vi "RS 485 COM In.vi"(8 "error in":errorcluster, 11 "9871 COM In":T1={"Data"=[0, 0, 0, 0, 0, 0, 0, 0, 0, 0, 0, 0, 0, 0, 0, 0, 0, 0, 0, 0, 0, 0, 0, 0, 0, 0, 0, 0, 0, 0], "NumBytes"=0, "Port"=enum."Port 1", "Wait for Reply"=FALSE}) -> (0 "error IO":errorcluster, 3 "9871 COM Out":T1={"Data"=[0, 0, 0, 0, 0, 0, 0, 0, 0, 0, 0, 0, 0, 0, 0, 0, 0, 0, 0, 0, 0, 0, 0, 0, 0, 0, 0, 0, 0, 0], "NumBytes"=0, "Port"=enum."Port 1", "Wait for Reply"=FALSE})   [LabVIEW 2015]
uses:
  <vilib>/eio/EIOMethodNode/EIOMethodNode.xnode
  <vilib>/rvi/eio/common/nirviEmuTemplateMethod_errors.vi
  Port Selector.ctl
  9871 COM In.ctl
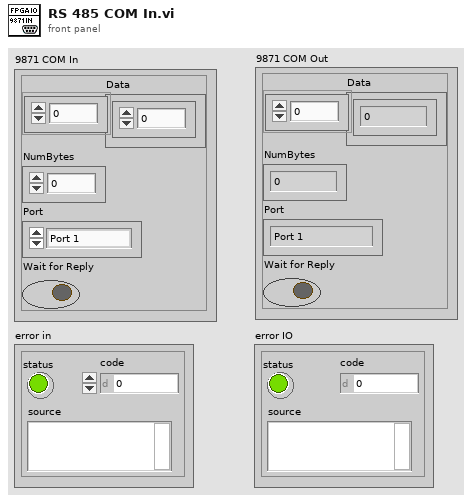
[diagram p1: front panel]
types:
  T1 = typedef "9871 COM In.ctl" = cluster{"Data":u8[], "NumBytes":i32, "Port":T2, "Wait for Reply":bool}
  T2 = typedef "Port Selector.ctl" = enum16{"Port 1", "Port 2", "Port 3", "Port 4", "None"}
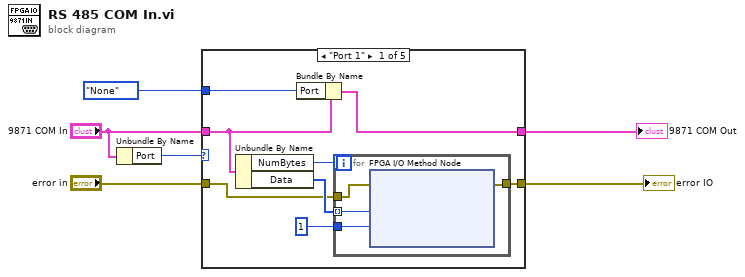
[diagram p0: block diagram]
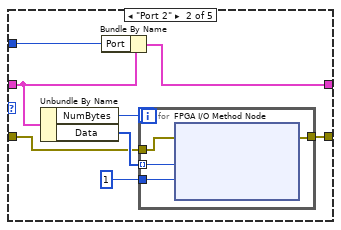
[diagram p2: hidden frame]
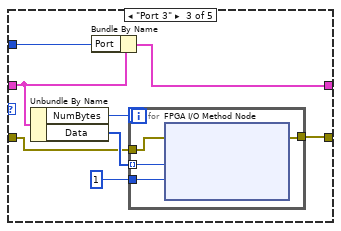
[diagram p3: hidden frame]
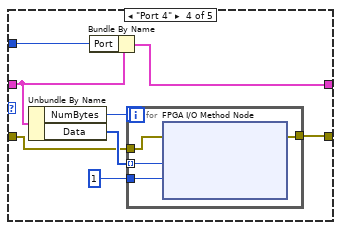
[diagram p4: hidden frame]
diagram:
  n1 = Unbundle By Name("9871 COM In") -> ("Port"=w2:T2)
  n2 = case shown="\"Port 1\"" w2 {
    tunnel: "9871 COM In" -> [w10 w26 w33 w46 w56]
    tunnel: [w11 w23 w35 w47 w56] -> w5
    tunnel: "error in" -> [w9 w22 w34 w45 w55]
    tunnel: [w8 w20 w32 w44 w55] -> w3
    tunnel: Port_Selector."None" ("Port") -> [w7 w19 w31 w43 _]
    frame "Port 1" {
      n3 = Unbundle By Name(w10) -> ("NumBytes"=w14:i32, "Data"=w13:u8[])
      n4 = Bundle By Name(cluster=w10, "Port"=w7) -> (w11:T1)
      n5 = for {
        N: w14 -> [_]
        tunnel: w13 -> [w18] mode=indexing
        tunnel: [w17] -> w8
        tunnel: w9 -> [w16]
        tunnel: 1 ("Timeout (ms)") -> [w15]
        n6 = xnode "FPGA I/O Method Node"("error in"=w16, "Data"=w18, "Timeout (ms)"=w15) -> ("error out"=w17:errorcluster)  [unwired: 1 in, 2 out]
      }
    }
    frame "Port 2" {
      n7 = Unbundle By Name(w26) -> ("NumBytes"=w25:i32, "Data"=w24:u8[])
      n8 = Bundle By Name(cluster=w26, "Port"=w19) -> (w23:T1)
      n9 = for {
        N: w25 -> [_]
        tunnel: w24 -> [w30] mode=indexing
        tunnel: [w29] -> w20
        tunnel: w22 -> [w28]
        tunnel: 1 ("Timeout (ms)") -> [w27]
        n10 = xnode "FPGA I/O Method Node"("error in"=w28, "Data"=w30, "Timeout (ms)"=w27) -> ("error out"=w29:errorcluster)  [unwired: 1 in, 2 out]
      }
    }
    frame "Port 3" {
      n11 = Unbundle By Name(w33) -> ("NumBytes"=w38:i32, "Data"=w37:u8[])
      n12 = Bundle By Name(cluster=w33, "Port"=w31) -> (w35:T1)
      n13 = for {
        N: w38 -> [_]
        tunnel: w37 -> [w42] mode=indexing
        tunnel: [w41] -> w32
        tunnel: w34 -> [w40]
        tunnel: 1 ("Timeout (ms)") -> [w39]
        n14 = xnode "FPGA I/O Method Node"("error in"=w40, "Data"=w42, "Timeout (ms)"=w39) -> ("error out"=w41:errorcluster)  [unwired: 1 in, 2 out]
      }
    }
    frame "Port 4" {
      n15 = Unbundle By Name(w46) -> ("NumBytes"=w50:i32, "Data"=w49:u8[])
      n16 = Bundle By Name(cluster=w46, "Port"=w43) -> (w47:T1)
      n17 = for {
        N: w50 -> [_]
        tunnel: w49 -> [w54] mode=indexing
        tunnel: [w53] -> w44
        tunnel: w45 -> [w52]
        tunnel: 1 ("Timeout (ms)") -> [w51]
        n18 = xnode "FPGA I/O Method Node"("error in"=w52, "Data"=w54, "Timeout (ms)"=w51) -> ("error out"=w53:errorcluster)  [unwired: 1 in, 2 out]
      }
    }
    frame "None", Default {
    }
  }
  "9871 COM Out" <- w5
  "error IO" <- w3
